vi "Add Fixed Wheel.vi"(8 "error in (no error)":errorcluster, 10 "wheel name":string, 11 "steering frame ref in":refnum<data-value>) -> (0 "error out":errorcluster, 1 "active wheel indexes out":i32[](array[numeric]), 3 "steering frame ref out":refnum<data-value>)   [LabVIEW 2017, in "NI_Robotics_Configure Steering Frame.lvlib"]
uses:
  <vilib>/robotics/Dialog/Configure Steering Frame/NI_Robotics_Configure Steering Frame.lvlib
  <vilib>/robotics/Steering/Steering Frame/NI_Robotics_Steering Frame.lvclass
  <vilib>/robotics/Steering/Wheel/Wheel Parameters.ctl
  <vilib>/robotics/Steering/Wheel/Rotation Direction.ctl
  <vilib>/robotics/Steering/Steering Frame/NI_Robotics_Steering Frame.lvclass/NI_Robotics_Steering Frame.ctl
  <vilib>/robotics/Steering/Fixed Wheel/NI_Robotics_Fixed Wheel.lvclass
  c:/Program Files (x86)/National Instruments/LabVIEW 2017/vi.lib/robotics/Steering/Wheel/NI_Robotics_Wheel.lvclass
  <vilib>/robotics/Steering/Wheel/NI_Robotics_Wheel.lvclass
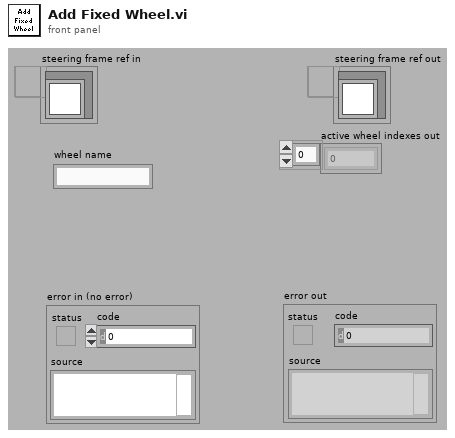
[diagram p1: front panel]
types:
  T1 = typedef "NI_Robotics_Wheel.lvclass/Wheel Parameters.ctl" = cluster{"wheel radius":dbl, "gear ratio":dbl, "forward rotation direction":T2}
  T2 = typedef "NI_Robotics_Wheel.lvclass/Rotation Direction.ctl" = u16
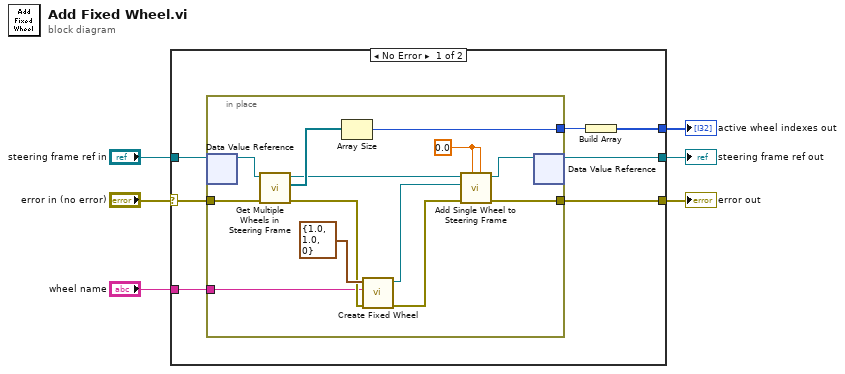
[diagram p0: block diagram]
diagram:
  n1 = case shown="No Error" "error in (no error)" {
    selector: "error in (no error)" -> [w13 w28]
    tunnel: [w12 w28] -> w5
    tunnel: "steering frame ref in" -> [w11 w27]
    tunnel: [w10 w27] -> w4
    tunnel: [w8 _] -> w3
    tunnel: "wheel name" -> [w7 _]
    frame No Error {
      n2 = in-place {
        in-place-border: w13 -> [w16]
        in-place-border: [w25] -> w9
        in-place-border: [w21] -> w12
        in-place-border: w7 -> [w14]
        w20 = 0.0 ("y position")
        n3 = in-place-dvr #1(w11) -> (w18:refnum<class "NI_Robotics_Steering Frame.lvclass">)  [unwired: 1 out]
        n4 = call <vilib>:"Get Multiple Wheels in Steering Frame.vi"("error in (no error)"=w16, "steering frame in"=w18) -> ("error out"=w15:errorcluster, "wheels"=w19:refnum<class "NI_Robotics_Wheel.lvclass">[], "steering frame out"=w17:refnum<class "NI_Robotics_Steering Frame.lvclass">)  [unwired: 3 in, 4 out]
        n5 = Array Size(array=w19) -> (size(s)=w25:i32)
        n6 = call <vilib>:"Create Fixed Wheel.vi"("error in (no error)"=w15, "wheel name"=w14, "wheel parameters"=T1 {"wheel radius"=1.0, "gear ratio"=1.0, "forward rotation direction"=0}) -> ("error out"=w24:errorcluster, "fixed wheel out"=w23:refnum<class "NI_Robotics_Fixed Wheel.lvclass">)  [unwired: 7 in]
        n7 = call <vilib>:"Add Single Wheel to Steering Frame.vi"("x position"=w20, "y position"=w20, "error in (no error)"=w24, "wheel"=w23, "steering frame in"=w17) -> ("error out"=w21:errorcluster, "steering frame out"=w22:refnum<class "NI_Robotics_Steering Frame.lvclass">)  [unwired: 5 in]
        n8 = in-place-dvr #1(w22) -> (w10:refnum<data-value>)  [unwired: 1 out]
      }
      n9 = Build Array(w9) -> (w8:i32[])
    }
    frame Error {
    }
  }
  "error out" <- w5
  "active wheel indexes out" <- w3
  "steering frame ref out" <- w4
